vi "close data logs.vi"(8 "error in":errorcluster, 10 "Data":sgl[](array[numeric]), 11 "Ref file Data":refnum<file>[](array[refnum])) -> (0 "error out":errorcluster)   [LabVIEW 2015]
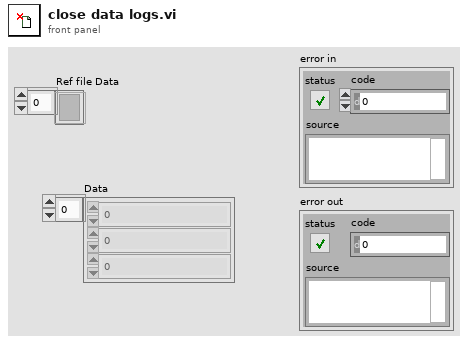
[diagram p1: front panel]
types:
  T1 = enum16{"big-endian, network order", "native, host order", "little-endian"}
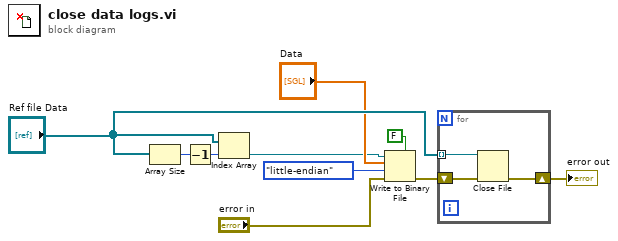
[diagram p0: block diagram]
diagram:
  n1 = Array Size(array="Ref file Data") -> (size(s)=w4:i32)
  n2 = Decrement(x=w4) -> (x-1=w3:i32)
  n3 = Index Array(array="Ref file Data", index=w3) -> (element=w7:refnum<file>)
  n4 = Write to Binary File(file (use dialog)=w7, data="Data", error in="error in", 5:FALSE ("prepend array or string size? (T)"), 9:T1."little-endian" ("byte order (0:big-endian, network order)")) -> (error out=w10:errorcluster)  [unwired: 3 out]
  n5 = for {
    shift-right: [w13] -> w2
    shift-left: w10 -> [w12]
    tunnel: "Ref file Data" -> [w11] mode=indexing
    n6 = Close File(refnum=w11, error in=w12) -> (error out=w13:errorcluster)  [unwired: 1 out]
  }
  "error out" <- w2
